vi "hexapod_server.vi"() -> ()   [LabVIEW 2011]
panel:
  out "Axes":string[](array[string])=["X", "Y", "Z", "U", "V", "W"]
  out "Position":dbl[](array[numeric])
  out "Ready":bool
  out "Pivot point":dbl[](array[numeric])
  in  "stop":bool
  out "Move possible":bool
  in  "Velocity":dbl=2.0
  out "Identification":string
  out "Hexapod initialized?":bool
  # "HEXAPOD server"
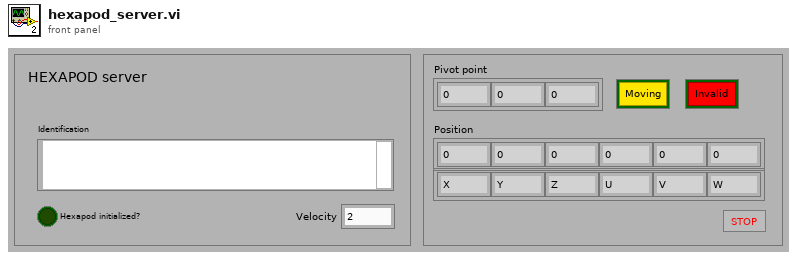
[diagram p1: front panel]
types:
  T1 = cluster{"Array of Double[0]":dbl, "Array of Double[1]":dbl, "Array of Double[2]":dbl}
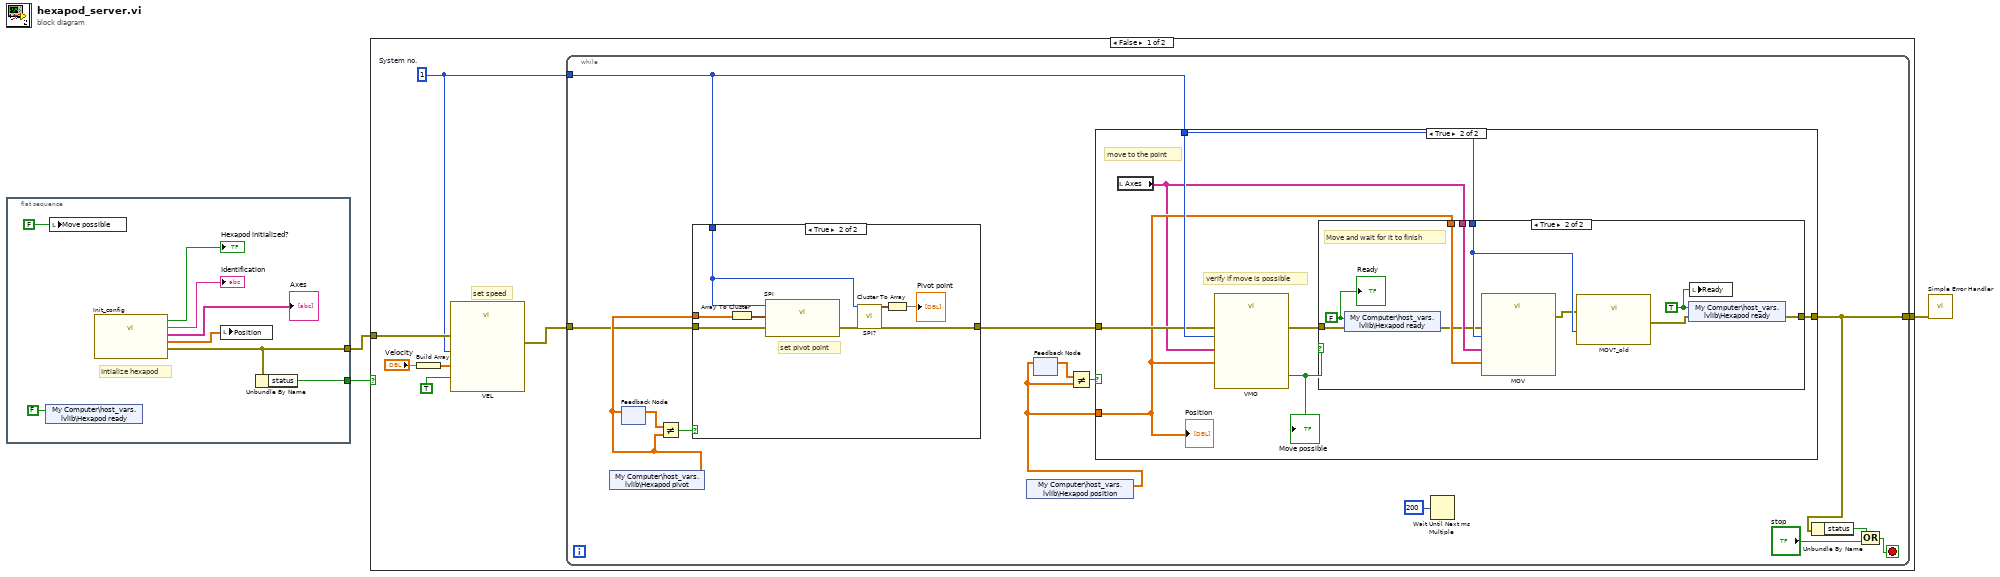
[diagram p0: block diagram]
diagram:
  n1 = flat-sequence {
    tunnel: [w8] -> w3
    tunnel: [w7] -> w2
    frame #0 {
      # "Intialize hexapod"
      n2 = shared-variable "My Computer\\host_vars.lvlib\\Hexapod ready"(FALSE ("Hexapod ready")) -> ()  [unwired: 1 in, 1 out]
      n3 = local write "Move possible"(FALSE ("Move possible")) -> ()
      n4 = call "Init_config.vi"() -> ("Hexapod initialized?"=→"Hexapod initialized?":bool, "Identification"=→"Identification":string, "Conn. Axes"=→"Axes":string[], "Position"=w5:dbl[], "error out"=w8:errorcluster)  [unwired: 11 in]
      n5 = local write "Position"(w5) -> ()
      n6 = Unbundle By Name(w8) -> ("status"=w7:bool)
    }
  }
  n7 = case shown="False" w2 {
    tunnel: w3 -> [w17 w61]
    tunnel: [w12 w61] -> w1
    frame False {
      w16 = 1  # System no.
      # "set speed"
      n8 = Build Array("Velocity") -> (w13:dbl[])
      n9 = call "VEL.vi"("System no."=w16, "Velocity values"=w13, "error in"=w17, "Without axis ID?"=TRUE) -> ("error out"=w15:errorcluster)  [unwired: 14 in, 1 out]
      n10 = while {
        tunnel: w16 -> [w26]
        tunnel: w15 -> [w25]
        tunnel: [w21] -> w12
        stop <- w22 stop-if-true
        n11 = shared-variable "My Computer\\host_vars.lvlib\\Hexapod pivot"() -> (w32:dbl[])  [unwired: 1 in, 1 out]
        n12 = feedback #1() -> (w29:dbl[])  [unwired: 1 in]
        n13 = feedback-in #1(w32) -> ()
        n14 = Not Equal?(x=w29, y=w32) -> (x != y?=w28:bool)
        n15 = case shown="True" w28 {
          tunnel: w26 -> [_ w38]
          tunnel: w32 -> [_ w36]
          tunnel: [w33 w35] -> w27
          tunnel: w25 -> [w33 w34]
          frame False {
          }
          frame True {
            # "set pivot point"
            n16 = Array To Cluster(array=w36) -> (cluster=w37:T1)
            n17 = call "SPI.vi"("System no."=w38, "Pivot point coordinates"=w37, "error in"=w34) -> ("error out"=w41:errorcluster)  [unwired: 15 in, 1 out]
            n18 = call "SPI?.vi"("System no."=w38, "error in"=w41) -> ("Pivot point coordinates"=w39:cluster{"R":dbl, "S":dbl, "T":dbl}, "error out"=w35:errorcluster)  [unwired: 16 in]
            n19 = Cluster To Array(cluster=w39) -> (array=→"Pivot point":dbl[])
          }
        }
        n20 = shared-variable "My Computer\\host_vars.lvlib\\Hexapod position"() -> (w20:dbl[])  [unwired: 1 in, 1 out]
        n21 = feedback #2() -> (w30:dbl[])  [unwired: 1 in]
        n22 = feedback-in #2(w20) -> ()
        n23 = Not Equal?(x=w30, y=w20) -> (x != y?=w31:bool)
        n24 = case shown="True" w31 {
          tunnel: [w42 w48] -> w21
          tunnel: w26 -> [_ w46]
          tunnel: w20 -> [_ w44]
          tunnel: w27 -> [w42 w45]
          frame False {
          }
          frame True {
            # "move to the point"
            # "verify if move is possible"
            n25 = local read "Axes"() -> (w43:string[])
            n26 = call "VMO.vi"("System no."=w46, "Axes to command"=w43, "Position values"=w44, "error in"=w45) -> ("Move possible"=w47:bool, "error out"=w49:errorcluster)  [unwired: 14 in]
            "Move possible" <- w47
            n27 = case shown="True" w47 {
              tunnel: w49 -> [w50 w56]
              tunnel: w46 -> [_ w58]
              tunnel: w43 -> [_ w60]
              tunnel: [w50 w53] -> w48
              tunnel: w44 -> [_ w59]
              frame False {
              }
              frame True {
                w51 = TRUE ("Hexapod ready")
                w52 = FALSE ("Hexapod ready")
                # "Move and wait for it to finish"
                n28 = shared-variable "My Computer\\host_vars.lvlib\\Hexapod ready"(w52, error in=w56) -> (error out=w55:errorcluster)
                n29 = call "MOV.vi"("System no."=w58, "Axes to move"=w60, "Position values"=w59, "error in"=w55) -> ("error out"=w57:errorcluster)  [unwired: 15 in]
                n30 = call "MOV?_old.vi"("System no."=w58, "error in"=w57) -> ("error out"=w54:errorcluster)  [unwired: 16 in, 1 out]
                n31 = shared-variable "My Computer\\host_vars.lvlib\\Hexapod ready"(w51, error in=w54) -> (error out=w53:errorcluster)
                n32 = local write "Ready"(w51) -> ()
                "Ready" <- w52
              }
            }
            "Position" <- w44
          }
        }
        n33 = Wait Until Next ms Multiple(millisecond multiple=u32 200) -> ()  [unwired: 1 out]
        n34 = Unbundle By Name(w21) -> ("status"=w24:bool)
        n35 = Compound Arithmetic op=OR(w24, "stop") -> (w22:bool)
      }
    }
    frame True {
      # "Initialization failed"
    }
  }
  n36 = call <vilib>:"Simple Error Handler.vi"("error in (no error)"=w1) -> ()  [unwired: 4 in, 5 out]
